vi "read single param.vi"(8 "error in (no error)":errorcluster, 10 "address":u16=401 format="%.0x", 11 "Stepper in":refnum<class "Stepper.lvclass">) -> (0 "error out":errorcluster, 2 "register":u16, 3 "Stepper out":refnum<class "Stepper.lvclass">)   [LabVIEW 2025, in "Stepper.lvclass"]
uses:
  Stepper.lvclass
  Stepper.lvclass/Stepper.ctl
  <vilib>/NI/Modbus Library/API/Master/Modbus Master.lvclass
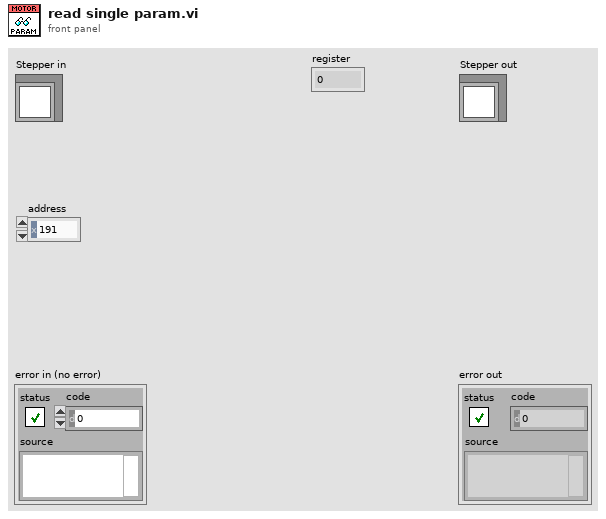
[diagram p1: front panel]
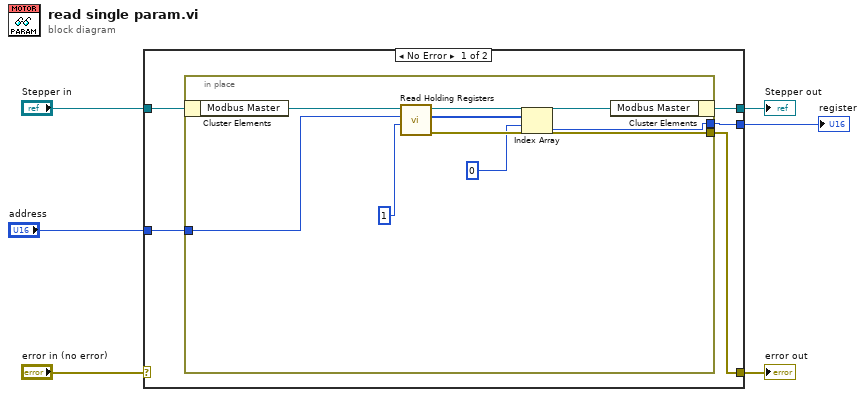
[diagram p0: block diagram]
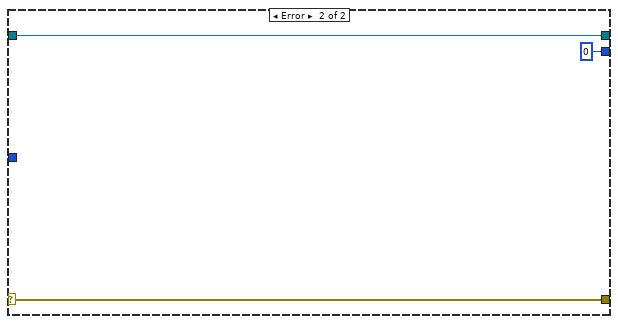
[diagram p2: hidden frame]
diagram:
  n1 = case shown="No Error" "error in (no error)" {
    selector: "error in (no error)" -> [_ w22]
    tunnel: [w10 w22] -> w5
    tunnel: [w8 w21] -> w3
    tunnel: "Stepper in" -> [w11 w21]
    tunnel: "address" -> [w9 _]
    tunnel: [w7 u16 0 ("register")] -> w1
    frame No Error {
      n2 = in-place {
        in-place-border: [w18] -> w10
        in-place-border: w9 -> [w16]
        in-place-border: [w12] -> w7
        n3 = in-place-cluster #1(w11) -> ("Modbus Master"=w19:refnum<class "Modbus Master.lvclass">)
        n4 = call-dynamic "Read Holding Registers.vi"("number of inputs"=u16 1, "starting address"=w16, "Modbus master in"=w19) -> ("error out"=w18:errorcluster, "register values"=w14:u16[], "Modbus master out"=w15:refnum<class "Modbus Master.lvclass">)  [unwired: 6 in]
        n5 = Index Array(array=w14, index=0) -> (element=w12:u16)
        n6 = in-place-cluster #1("Modbus Master"=w15) -> (w8:refnum<class "Stepper.lvclass">)
      }
    }
    frame Error {
    }
  }
  "error out" <- w5
  "Stepper out" <- w3
  "register" <- w1
